vi "FileIO - Default for System Parameters.vi"() -> (3 "Sys Parameters":T1={"Results FilePath"=path "", "Analysis Parameters"={"Area"={"Lower Value"=0.0, "Upper Value"=0.0}, "Circle Filter Radius"={"Lower Value"=0.0, "Upper Value"=0.0}, "Edge Detection Threshold"=50}, "ROI Parameters"={"ROI size (in Radius)"={"Width"=1.0, "Height"=0.5}}})   [LabVIEW 2014]
uses:
  Custom Controls/TypeDef - System Configuration.ctl
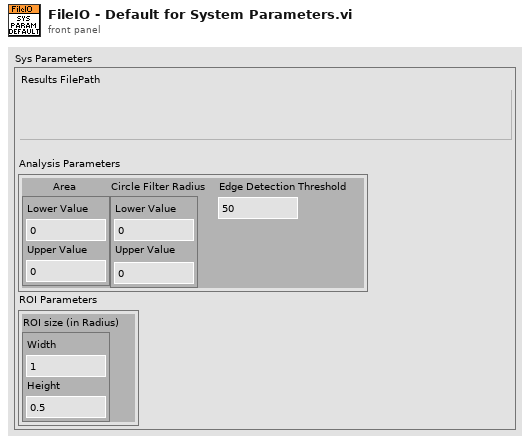
[diagram p1: front panel]
types:
  T1 = typedef "TypeDef - System Configuration.ctl" = cluster{"Results FilePath":path, "Analysis Parameters":cluster{"Area":cluster{"Lower Value":dbl, "Upper Value":dbl}, "Circle Filter Radius":cluster{"Lower Value":sgl, "Upper Value":sgl}, "Edge Detection Threshold":u16}, "ROI Parameters":cluster{"ROI size (in Radius)":cluster{"Width":dbl, "Height":dbl}}}
  T2 = cluster{"ROI size (in Radius)":cluster{"Width":dbl, "height":dbl}}
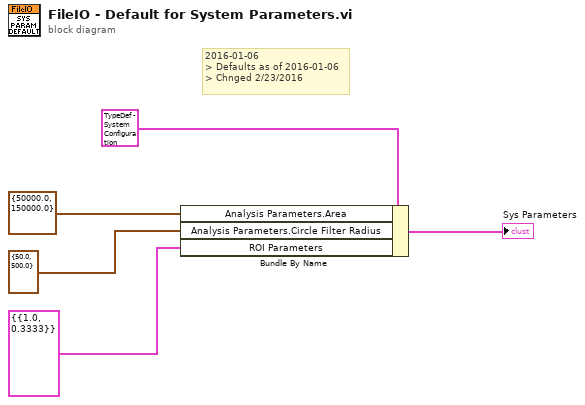
[diagram p0: block diagram]
diagram:
  # "2016-01-06\n> Defaults as of 2016-01-06\n> Chnged 2/23/2016"
  n1 = Bundle By Name(cluster=T1 {"Results FilePath"=path "", "Analysis Parameters"={"Area"={"Lower Value"=0.0, "Upper Value"=0.0}, "Circle Filter Radius"={"Lower Value"=0.0, "Upper Value"=0.0}, "Edge Detection Threshold"=50}, "ROI Parameters"={"ROI size (in Radius)"={"Width"=0.0, "Height"=0.0}}} ("Sys Parameters"), "Analysis Parameters.Area"=cluster{"Lower Value":dbl, "Upper Value":dbl} {"Lower Value"=50000.0, "Upper Value"=150000.0} ("Feret Filter"), "Analysis Parameters.Circle Filter Radius"=cluster{"Lower Value":sgl, "Upper Value":sgl} {"Lower Value"=50.0, "Upper Value"=500.0} ("Circle Filter Diameter"), "ROI Parameters"=T2 {"ROI size (in Radius)"={"Width"=1.0, "height"=0.3333}}) -> (→"Sys Parameters":T1)
